vi "Run Survey Plot (SubVI).vi"(6 "Folder to Save":string, 8 "Show terminal?":bool=TRUE, 9 "Survey csv":string, 10 "Ideal csv":string, 11 "Working Directory to Python scripts":path) -> (3 "standard error":string)   [LabVIEW 2016]
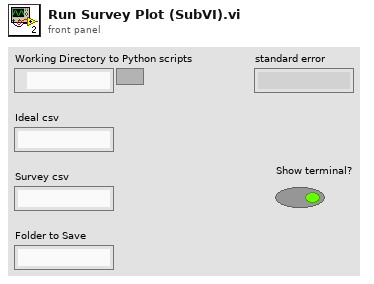
[diagram p1: front panel]
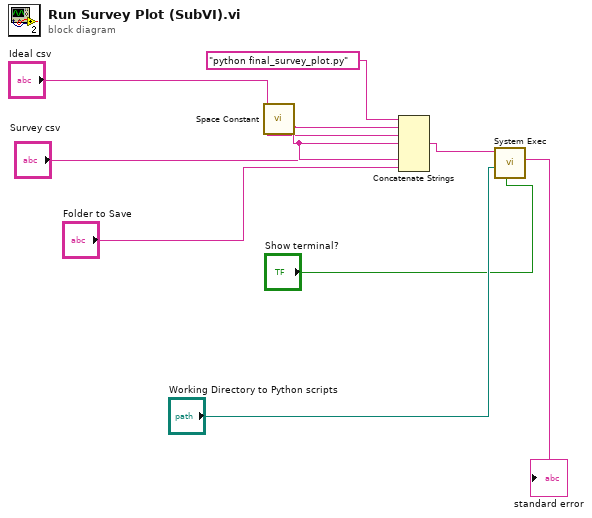
[diagram p0: block diagram]
diagram:
  n1 = call <vilib>:"Space Constant.vi"() -> ("String"=w6:string)
  n2 = Concatenate Strings("python final_survey_plot.py", w6, "Ideal csv", w6, "Survey csv", w6, "Folder to Save") -> (w7:string)
  n3 = call <vilib>:"System Exec.vi"("run minimized? (F)"="Show terminal?", "working directory"="Working Directory to Python scripts", "command line"=w7) -> ("standard error"=→"standard error":string)  [unwired: 5 in, 3 out]
